vi "Mean_of_10.vi"(11 "MeasMean0":dbl) -> (3 "mean":dbl)   [LabVIEW 2018]
uses:
  <vilib>/Analysis/baseanly.llb/Mean (DBL).vi
  <vilib>/Analysis/NI_AALBase.lvlib
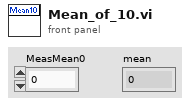
[diagram p1: front panel]
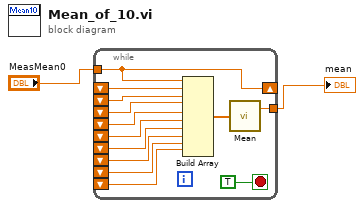
[diagram p0: block diagram]
diagram:
  n1 = while {
    shift-right: [w6] -> _
    shift-left: _ -> [w15]
    shift-left: _ -> [w14]
    shift-left: _ -> [w13]
    shift-left: _ -> [w12]
    shift-left: _ -> [w11]
    shift-left: _ -> [w10]
    shift-left: _ -> [w9]
    shift-left: _ -> [w8]
    shift-left: _ -> [w7]
    tunnel: "MeasMean0" -> [w6]
    tunnel: [w4] -> w2
    stop <- TRUE stop-if-true
    n2 = Build Array(w6, w15, w14, w13, w12, w11, w10, w9, w8, w7) -> (w5:dbl[])
    n3 = call-poly <vilib>:"Mean.vi"("X"=w5) -> ("mean"=w4:dbl)  [unwired: 1 out]
  }
  "mean" <- w2
